vi "压力数据保存判定.vi"(7 "路径":path, 8 "error in (no error)":errorcluster caption="错误输入（无错误）", 9 "布尔":bool, 11 "添加的数组":dbl[](array[numeric])) -> (0 "error out":errorcluster)   [LabVIEW 2017]
uses:
  <vilib>/Utility/file.llb/Write Delimited Spreadsheet (string).vi
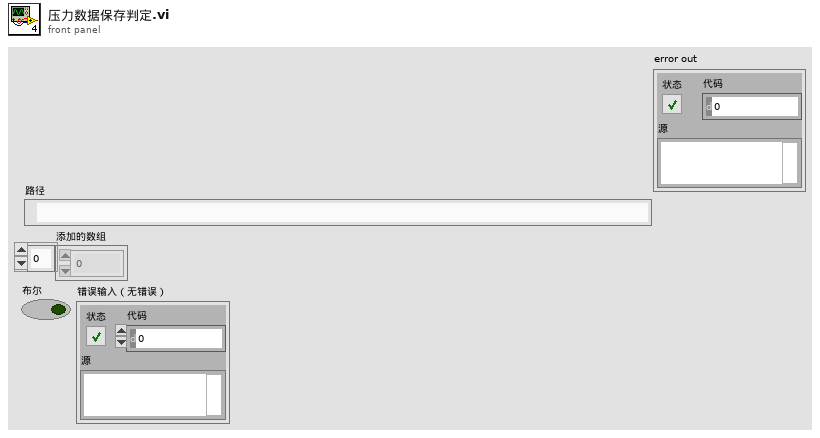
[diagram p1: front panel]
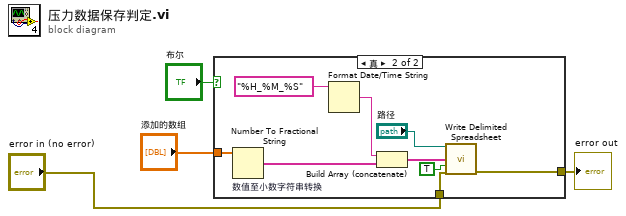
[diagram p0: block diagram]
diagram:
  n1 = case shown="真" "布尔" {
    tunnel: "添加的数组" -> [_ w11]
    tunnel: [w5 w7] -> w2
    tunnel: "error in (no error)" -> [w5 w6]
    frame False {
    }
    frame True {
      n2 = Number To Fractional String "数值至小数字符串转换"(number=w11) -> (F-format string=w10:string[])  [unwired: 3 in]
      n3 = Format Date/Time String(time format string (%c)="%H_%M_%S" ("时间格式字符串(%c)")) -> (date/time string=w12:string)  [unwired: 2 in]
      n4 = Build Array (concatenate)(w12, w10) -> (w9:string[])
      n5 = call-poly <vilib>:"Write Delimited Spreadsheet.vi"("file path (dialog if empty)"="路径", "1D data"=w9, "append to file? (new file:F)"=TRUE, "error in (no error)"=w6) -> ("error out"=w7:errorcluster)  [unwired: 10 in, 1 out]
    }
  }
  "error out" <- w2
